vi "Get Manager.vi"(9 "error in (no error)":errorcluster) -> (1 "error out":errorcluster, 3 "Subpanel.Edit":refnum<class "Subpanel.Edit.lvclass">)   [LabVIEW 2019, in "Subpanel.Edit.lvclass"]
uses:
  Subpanel.Edit.lvclass
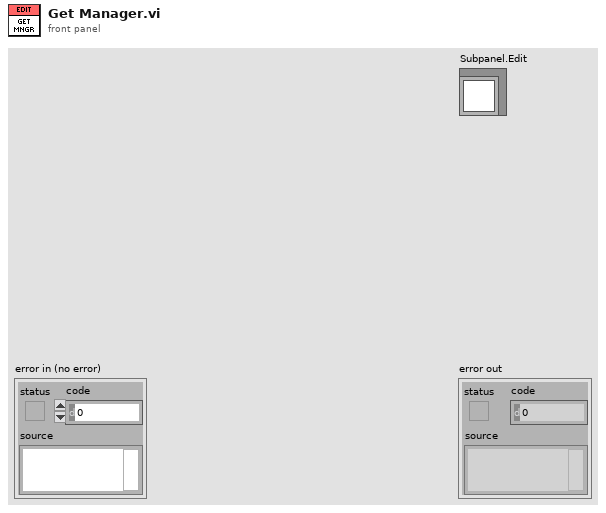
[diagram p1: front panel]
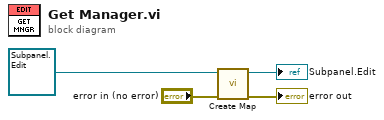
[diagram p0: block diagram]
diagram:
  n1 = call-dynamic "Create Map.vi"("error in (no error)"="error in (no error)", "Edit.Subpanel in"=refnum<class "Subpanel.Edit.lvclass"> refnum ("Subpanel.Edit out")) -> ("error out"=→"error out":errorcluster, "Edit.Subpanel out"=→"Subpanel.Edit":refnum<class "Subpanel.Edit.lvclass">)  [unwired: 8 in]
